vi "Marker Draw and Commands Loop.vi"(7 "Options":T1={"Color"=16723218, "pen"={"Width"=2, "Style"=enum."Solid"}, "font"={"Font Name"="Arial", "Size"=14, "Strikeout?"=FALSE, "Italic?"=FALSE, "Underline?"=FALSE, "Outline?"=FALSE, "Shadow?"=FALSE, "Bold?"=FALSE, "FontColor"=6908265}, "caption"="Click to set a point marker"}, 10 "XY Graph":refnum<vi>) -> ()   [LabVIEW 2015]
uses:
  controls/MarkerOptions.ctl
  subVIs/MarkersDVRType.ctl
  controls/markerType.ctl
  controls/GraphExt-Cmds.ctl
  controls/commands.ctl
  <vilib>/Utility/miscctls.llb/LVPoint32TypeDef.ctl
  controls/cmd_options.ctl
  controls/Simple Global for Marker Options.vi
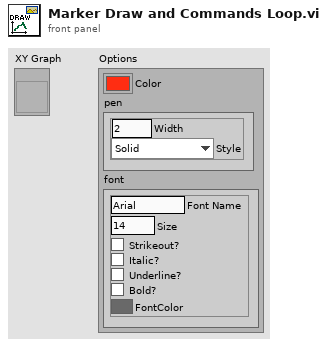
[diagram p1: front panel]
types:
  T1 = typedef "MarkerOptions.ctl" = cluster{"Color":u32, "pen":cluster{"Width":u16, "Style":enum32{"Solid", "Dash", "Dot", "DashDot", "DashDotDot"}}, "font":cluster{"Font Name":string, "Size":i16, "Strikeout?":bool, "Italic?":bool, "Underline?":bool, "Outline?":bool, "Shadow?":bool, "Bold?":bool, "FontColor":u32}, "caption":string}
  T2 = typedef "MarkersDVRType.ctl" = cluster{"Type":T3, "X":dbl, "Y":dbl, "X2":dbl, "Y2":dbl, "Text":string}
  T3 = typedef "markerType.ctl" = enum16{"point", "arrow", "horiz", "vert", "vert range", "horiz range", "box"}
  T4 = typedef "commands.ctl" = enum16{"up", "options", "click", "move", "type", "redraw"}
  T5 = typedef "LVPoint32TypeDef.ctl" = cluster{"Horizontal":i32, "Vertical":i32}
  T6 = cluster{"cmd":T4, "Type":T3, "Coords":T5, "Active Tool":i32, "mode":enum16{"drag", "none"}}
  T7 = typedef "GraphExt-Cmds.ctl" = cluster{"cmd":T4, "Type":T3, "Coords":T5, "text":string}
  T8 = typedef "cmd_options.ctl" = cluster{"Marker Color":u32, "Style":enum32{"Solid", "Dash", "Dot", "DashDot", "DashDotDot"}, "Width":u16, "Size":i16, "Color":u32}
  T9 = typedef "LVRectTypeDef.ctl" = cluster{"Left":i16, "Top":i16, "Right":i16, "Bottom":i16}
  T10 = enum32{"Solid", "Dash", "Dot", "DashDot", "DashDotDot"}
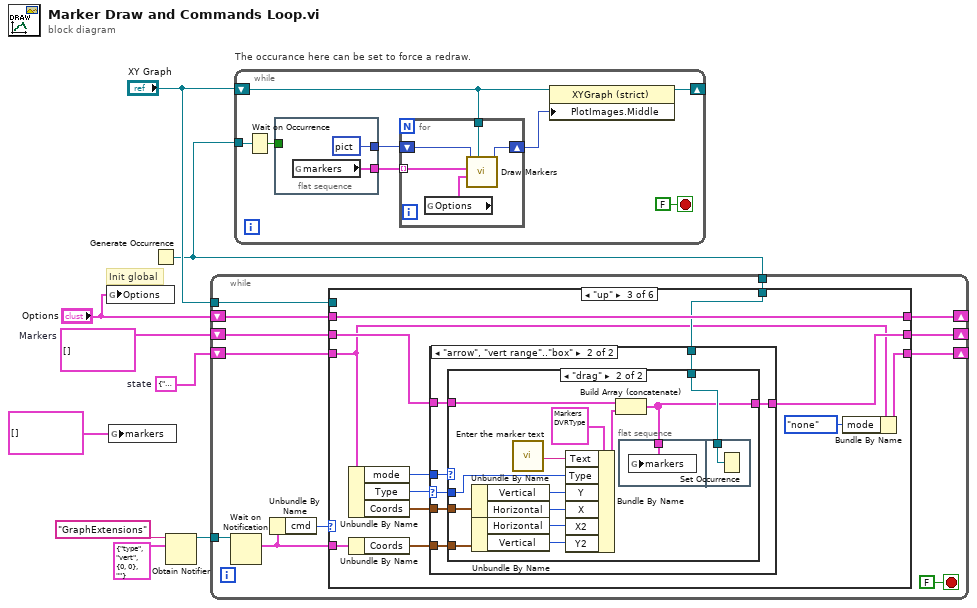
[diagram p0: block diagram]
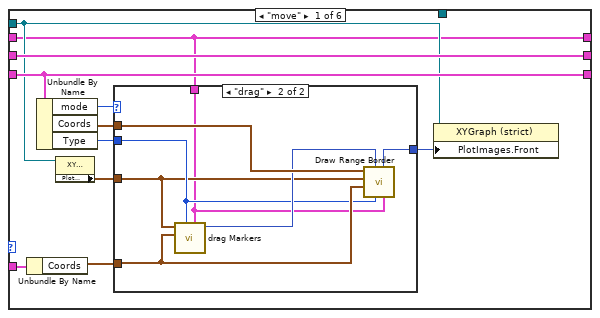
[diagram p2: hidden frame]
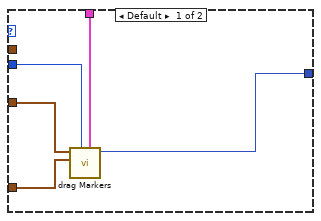
[diagram p3: hidden frame]
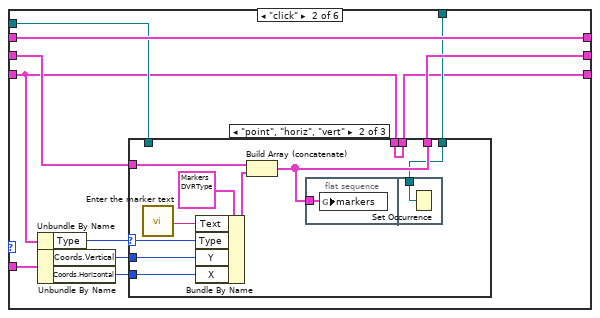
[diagram p4: hidden frame]
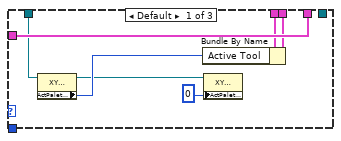
[diagram p5: hidden frame]
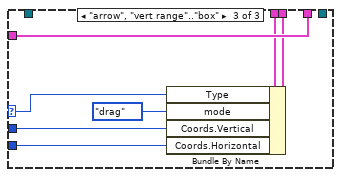
[diagram p6: hidden frame]
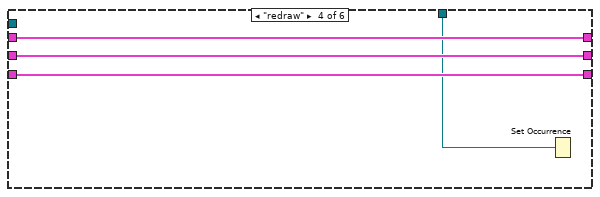
[diagram p9: hidden frame]
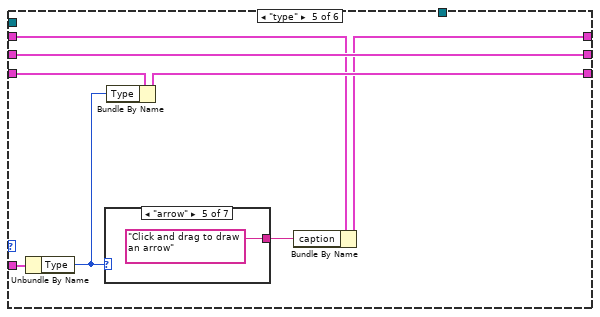
[diagram p10: hidden frame]
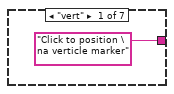
[diagram p11: hidden frame]
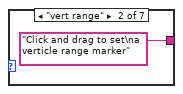
[diagram p12: hidden frame]
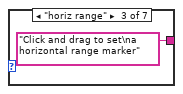
[diagram p13: hidden frame]
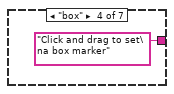
[diagram p14: hidden frame]
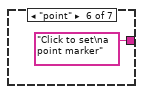
[diagram p15: hidden frame]
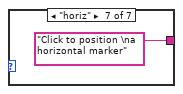
[diagram p16: hidden frame]
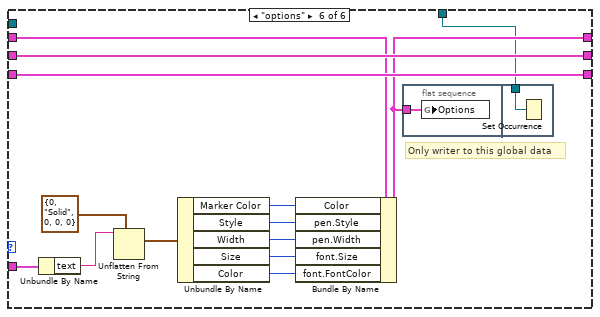
[diagram p17: hidden frame]
diagram:
  w5 = T6 {"cmd"=enum."click", "Type"=enum."point", "Coords"={"Horizontal"=0, "Vertical"=0}, "Active Tool"=0, "mode"=enum."none"}  # state
  w4 = T2[] []  # Markers
  # "Init global"
  # "The occurance here can be set to force a redraw."
  n1 = global write "Simple Global for Marker Options.vi" "Options"("Options") -> ()
  n2 = global write "Simple Global for Marker Options.vi" "markers"(T2[] [] ("appended array")) -> ()
  n3 = Generate Occurrence() -> (w3:refnum<k4>)
  n4 = Obtain Notifier(name (unnamed)="GraphExtensions", notification data type=T7 {"cmd"=enum."type", "Type"=enum."vert", "Coords"={"Horizontal"=0, "Vertical"=0}, "text"=""}) -> (notifier out=w8:refnum<notifier>)  [unwired: 2 in, 2 out]
  n5 = while {
    tunnel: w8 -> [w20]
    shift-right: [w16] -> _
    shift-left: "Options" -> [w17]
    shift-right: [w15] -> _
    shift-left: w4 -> [w14]
    shift-right: [w13] -> _
    shift-left: w5 -> [w12]
    tunnel: w3 -> [w11]
    tunnel: "XY Graph" -> [w10]
    stop <- FALSE stop-if-true
    n6 = Wait on Notification(notifier=w20) -> (notification=w19:T7)  [unwired: 3 in, 3 out]
    n7 = Unbundle By Name(w19) -> ("cmd"=w18:T4)
    n8 = case shown="\"up\"" w18 {
      tunnel: w17 -> [w22 w55 w93 w119 w123 w143]
      tunnel: w19 -> [w32 w54 w92 _ w128 w148]
      tunnel: [w22 w55 w93 w119 w122 w138] -> w16
      tunnel: [w31 w51 w86 w121 w129 w150] -> w15
      tunnel: w14 -> [w31 w47 w87 w121 w129 w150]
      tunnel: [w30 w48 w83 w120 w126 w149] -> w13
      tunnel: w12 -> [w30 w46 w84 w120 w127 w149]
      tunnel: w11 -> [_ w50 w85 w118 _ w137]
      tunnel: w10 -> [w24 w49 _ _ _ _]
      frame "move" {
        n9 = Unbundle By Name(w32) -> ("Coords"=w25:T5)
        n10 = Unbundle By Name(w30) -> ("mode"=w27:enum16{"drag", "none"}, "Coords"=w29:T5, "Type"=w26:T3)
        n11 = property on="Property Node" class="XYGraph (strict)"(reference=w24) -> ("Plot Bounds"=w23:T9)  [unwired: 1 in, 2 out]
        n12 = case shown="\"drag\"" w27 {
          tunnel: w29 -> [_ w44]
          tunnel: [w37 w43] -> w28
          tunnel: w22 -> [w36 w38]
          tunnel: w26 -> [w35 w40]
          tunnel: w25 -> [w34 w41]
          tunnel: w23 -> [w33 w39]
          frame Default {
            n13 = call "drag Markers.vi"("Marker Options"=w36, "Type"=w35, "Coords"=w34, "Plot Area Bounds"=w33) -> ("new picture"=w37:picture)  [unwired: 7 in]
          }
          frame "drag" {
            n14 = call "drag Markers.vi"("Marker Options"=w38, "Type"=w40, "Coords"=w41, "Plot Area Bounds"=w39) -> ("new picture"=w42:picture)  [unwired: 7 in]
            n15 = call "Draw Range Border.vi"("Marker Options"=w38, "Type"=w40, "picture"=w42, "end Coords"=w41, "Plot Bounds"=w39, "Start Coords"=w44) -> ("new picture"=w43:picture)  [unwired: 5 in]
          }
        }
        n16 = property on="Property Node" class="XYGraph (strict)"(reference=w24, "PlotImages.Front"=w28) -> ()  [unwired: 1 in, 2 out]
      }
      frame "click" {
        n17 = Unbundle By Name(w46) -> ("Type"=w45:T3)
        n18 = Unbundle By Name(w54) -> ("Coords.Vertical"=w53:i32, "Coords.Horizontal"=w52:i32)
        n19 = case shown="\"point\", \"horiz\", \"vert\"" w45 {
          selector: w45 -> [_ w65 w75]
          tunnel: w47 -> [w62 w71 w81]
          tunnel: w53 -> [_ w64 w77]
          tunnel: w52 -> [_ w69 w76]
          tunnel: [w62 w68 w81] -> w51
          tunnel: w50 -> [_ w63 _]
          tunnel: w49 -> [w61 _ _]
          tunnel: w46 -> [w60 w66 w80]
          tunnel: [w59 w66 w79] -> w48
          frame Default {
            n20 = property class="XYGraph (strict)"(reference=w61) -> (reference out=w57:refnum<vi>, "ActPaletteTool"=w58:i32)  [unwired: 1 in, 1 out]
            n21 = Bundle By Name(cluster=w60, "Active Tool"=w58) -> (w59:T6)
            n22 = property class="XYGraph (strict)"(reference=w57, "ActPaletteTool"=0 ("Palette:Active Tool")) -> ()  [unwired: 1 in, 2 out]
          }
          frame "point", "horiz", "vert" {
            n23 = call "Enter the marker text"() -> (17:w67:string)  [unwired: 17 in, 2 out]
            n24 = Bundle By Name(cluster=T2 {"Type"=enum."vert", "X"=2.0, "Y"=2.0, "X2"=2.0, "Y2"=2.0, "Text"="Drag and click to\nposition a marker"} ("Markers"), "Text"=w67, "Type"=w65, "Y"=w64, "X"=w69) -> (w70:T2)
            n25 = Build Array (concatenate)(w71, w70) -> (w68:T2[])
            n26 = flat-sequence {
              tunnel: w68 -> [w73]
              tunnel: w63 -> [w74]
              frame #0 {
                n27 = global write "Simple Global for Marker Options.vi" "markers"(w73) -> ()
              }
              frame #1 {
                n28 = Set Occurrence(w74) -> ()
              }
            }
          }
          frame "arrow", "vert range".."box" {
            n29 = Bundle By Name(cluster=w80, "Type"=w75, "mode"=enum16{"drag", "none"}."drag", "Coords.Vertical"=w77, "Coords.Horizontal"=w76) -> (w79:T6)
          }
        }
      }
      frame "up" {
        n30 = Unbundle By Name(w84) -> ("mode"=w88:enum16{"drag", "none"}, "Type"=w91:T3, "Coords"=w90:T5)
        n31 = Unbundle By Name(w92) -> ("Coords"=w89:T5)
        n32 = case shown="\"arrow\", \"vert range\"..\"box\"" w91 {
          selector: w91 -> [_ w100]
          tunnel: w90 -> [_ w96]
          tunnel: w89 -> [_ w97]
          tunnel: w88 -> [_ w101]
          tunnel: w87 -> [w94 w99]
          tunnel: [w94 w98] -> w86
          tunnel: w85 -> [_ w95]
          frame Default {
          }
          frame "arrow", "vert range".."box" {
            n33 = case shown="\"drag\"" w101 {
              tunnel: w100 -> [_ w105]
              tunnel: w99 -> [w102 w112]
              tunnel: [w102 w103] -> w98
              tunnel: w97 -> [_ w111]
              tunnel: w96 -> [_ w110]
              tunnel: w95 -> [_ w104]
              frame Default {
              }
              frame "drag" {
                n34 = Unbundle By Name(w110) -> ("Vertical"=w109:i32, "Horizontal"=w108:i32)
                n35 = Unbundle By Name(w111) -> ("Horizontal"=w107:i32, "Vertical"=w106:i32)
                n36 = call "Enter the marker text"() -> (17:w114:string)  [unwired: 17 in, 2 out]
                n37 = Bundle By Name(cluster=T2 {"Type"=enum."vert", "X"=2.0, "Y"=2.0, "X2"=2.0, "Y2"=2.0, "Text"="Drag and click to\nposition a marker"} ("Markers"), "Text"=w114, "Type"=w105, "Y"=w109, "X"=w108, "X2"=w107, "Y2"=w106) -> (w113:T2)
                n38 = Build Array (concatenate)(w112, w113) -> (w103:T2[])
                n39 = flat-sequence {
                  tunnel: w103 -> [w116]
                  tunnel: w104 -> [w117]
                  frame #0 {
                    n40 = global write "Simple Global for Marker Options.vi" "markers"(w116) -> ()
                  }
                  frame #1 {
                    n41 = Set Occurrence(w117) -> ()
                  }
                }
              }
            }
          }
        }
        n42 = Bundle By Name(cluster=w84, "mode"=enum16{"drag", "none"}."none") -> (w83:T6)
      }
      frame "redraw" {
        n43 = Set Occurrence(w118) -> ()
      }
      frame "type" {
        n44 = Unbundle By Name(w128) -> ("Type"=w125:T3)
        n45 = case shown="\"arrow\"" w125 {
          tunnel: ["Click to position \na verticle marker" ("Text") "Click and drag to set\na verticle range marker" ("Text") "Click and drag to set\na horizontal range marker" ("Text") "Click and drag to set\na box marker" ("Text") "Click and drag to draw an arrow" ("Text") "Click to set\na point marker" ("Text") "Click to position \na horizontal marker" ("Text")] -> w124
          frame "vert" {
          }
          frame "vert range" {
          }
          frame "horiz range" {
          }
          frame "box" {
          }
          frame "arrow" {
          }
          frame "point" {
          }
          frame "horiz" {
          }
        }
        n46 = Bundle By Name(cluster=w127, "Type"=w125) -> (w126:T6)
        n47 = Bundle By Name(cluster=w123, "caption"=w124) -> (w122:T1)
      }
      frame "options" {
        # "Only writer to this global data"
        n48 = Unbundle By Name(w148) -> ("text"=w147:string)
        n49 = Unflatten From String(type=T8 {"Marker Color"=0, "Style"=enum."Solid", "Width"=0, "Size"=0, "Color"=0} ("cluster"), binary string=w147) -> (value=w146:T8)  [unwired: 3 in, 2 out]
        n50 = Unbundle By Name(w146) -> ("Marker Color"=w144:u32, "Style"=w142:T10, "Width"=w141:u16, "Size"=w140:i16, "Color"=w139:u32)
        n51 = Bundle By Name(cluster=w143, "Color"=w144, "pen.Style"=w142, "pen.Width"=w141, "font.Size"=w140, "font.FontColor"=w139) -> (w138:T1)
        n52 = flat-sequence {
          tunnel: w138 -> [w151]
          tunnel: w137 -> [w152]
          frame #0 {
            n53 = global write "Simple Global for Marker Options.vi" "Options"(w151) -> ()
          }
          frame #1 {
            n54 = Set Occurrence(w152) -> ()
          }
        }
      }
    }
  }
  n55 = while {
    shift-right: [w154] -> _
    shift-left: "XY Graph" -> [w153]
    tunnel: w3 -> [w160]
    stop <- FALSE stop-if-true
    n56 = Wait on Occurrence(2:w160) -> (0:w156:bool)  [unwired: 2 in]
    n57 = flat-sequence {
      tunnel: [w161] -> w158
      tunnel: [picture data[5B] ("new picture")] -> w157
      tunnel: w156 -> [_]
      frame #0 {
        n58 = global read "Simple Global for Marker Options.vi" "markers"() -> (w161:T2[])
      }
    }
    n59 = for {
      tunnel: w158 -> [w167] mode=indexing
      shift-right: [w165] -> w159
      shift-left: w157 -> [w166]
      tunnel: w153 -> [w164]
      n60 = global read "Simple Global for Marker Options.vi" "Options"() -> (w163:T1)
      n61 = call "Draw Markers.vi"("XYGraph in"=w164, "Marker Options"=w163, "Marker"=w167, "picture"=w166) -> ("new picture"=w165:picture)  [unwired: 7 in]
    }
    n62 = property class="XYGraph (strict)"(reference=w153, "PlotImages.Middle"=w159) -> (reference out=w154:refnum<vi>)  [unwired: 1 in, 1 out]
  }
